vi "File Merge classes test.vi"   [LabVIEW 2017]
uses:
  Classes/FileMerge/FileMerge.lvclass
  Classes/Datalog/DataLog.lvclass
  C:/Users/Public/Documents/UCAR/APAR Board Test/LVSource/Classes/Datalog/DataLog.lvclass
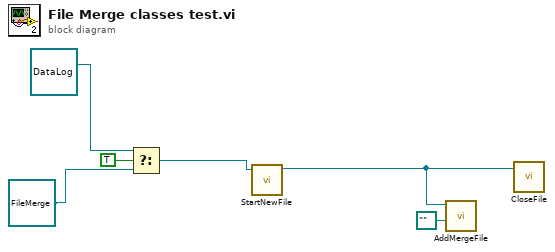
[diagram p0: block diagram]
diagram:
  n1 = Select(t=refnum<class "DataLog.lvclass"> refnum ("DataLog.lvclass"), s=TRUE, f=refnum<class "FileMerge.lvclass"> refnum ("FileMerge.lvclass")) -> (s? t:f=w3:refnum<class "DataLog.lvclass">)
  n2 = call-dynamic "StartNewFile.vi"("DataLog in"=w3) -> ("DataLog out"=w2:refnum<class "DataLog.lvclass">)  [unwired: 9 in, 1 out]
  n3 = call-dynamic "AddMergeFile.vi"("ExistingFilePath"=path "", "DataLog in"=w2) -> ()  [unwired: 8 in, 2 out]
  n4 = call-dynamic "CloseFile.vi"("DataLog in"=w2) -> ()  [unwired: 9 in, 2 out]
